vi "Get Is Valid.vi"(8 "error in (no error)":errorcluster, 11 "VariableContainer in":refnum<class "VariableContainer.lvclass">) -> (0 "error out":errorcluster, 2 "Valid?":bool, 3 "VariableContainer out":refnum<class "VariableContainer.lvclass">)   [LabVIEW 2020, in "HTS.lvlib" / "VariableContainer.lvclass"]
uses:
  VariableContainer.lvclass
  VariableContainer.lvclass/VariableContainer.ctl
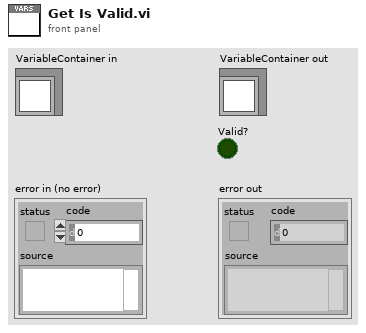
[diagram p1: front panel]
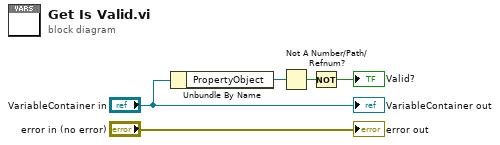
[diagram p0: block diagram]
diagram:
  n1 = Unbundle By Name("VariableContainer in") -> ("PropertyObject"=w3:refnum<k7>)
  n2 = Not A Number/Path/Refnum?(number/path/refnum=w3) -> (NaN/Path/Refnum?=w2:bool)
  n3 = Not(x=w2) -> (.not. x?=→"Valid?":bool)
  "error out" <- "error in (no error)"
  "VariableContainer out" <- "VariableContainer in"
